vi "vi ref test.vi"   [LabVIEW 2013]
types:
  T1 = typedef "Image Type" = u32
  T2 = typedef "IMAQ Image.ctl" = refnum<image>
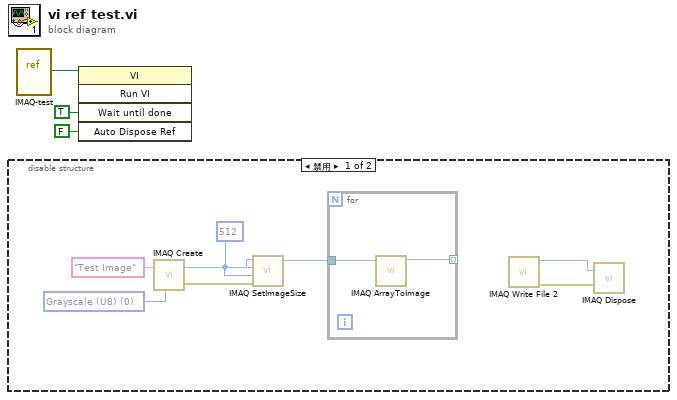
[diagram p0: block diagram]
diagram:
  n1 = disable-structure shown="禁用" {
    frame Disabled {
      w5 = T1 0 items=["Grayscale (U8)", "Grayscale (I16)", "Grayscale (SGL)", "Complex (CSG)", "RGB (U32)", "HSL (U32)", "RGB (U64)", "Grayscale (U16)"] ("Image Type")
      w7 = 512 ("X Resolution")
      n2 = call "IMAQ Create"("Image Name"="Test Image", "Image Type"=w5) -> ("New Image"=w8:T2, "error out"=w9:errorcluster)  [unwired: 3 in]
      n3 = call "IMAQ SetImageSize"("error in (no error)"=w9, "Y Resolution"=w7, "X Resolution"=w7, "Image"=w8) -> ("Image Out"=w4:T2)  [unwired: 1 in, 1 out]
      n4 = for {
        tunnel: w4 -> [w13]
        tunnel: [w12] -> _ mode=indexing
        n5 = call "IMAQ ArrayToImage"("Image"=w13) -> ("Image Out"=w12:T2)  [unwired: 9 in, 1 out]
      }
      n6 = call-poly "IMAQ Write File 2"() -> ("error out"=w10:errorcluster, "Image Out (duplicate)"=w11:T2)  [unwired: 10 in]
      n7 = call "IMAQ Dispose"("Image"=w11, "error in (no error)"=w10) -> ()  [unwired: 4 in, 1 out]
    }
    frame Enabled {
    }
  }
  n8 = vi-ref "IMAQ-test.vi"() -> (w3:refnum<vi>)
  n9 = invoke class="VI" method="Run VI"(reference=w3, "Wait until done"=TRUE ("结束前等待"), "Auto Dispose Ref"=FALSE ("自动销毁引用")) -> ()  [unwired: 2 in, 5 out]
